vi "ADIS16448 Loop Inc Acquire Count.vi"(8 "error in (no error)":errorcluster) -> (0 "error out":errorcluster)   [LabVIEW 2019]
uses:
  ADIS16448 Globals.vi
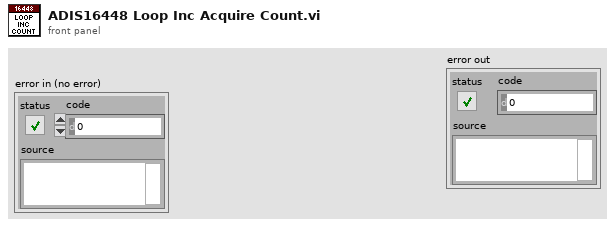
[diagram p1: front panel]
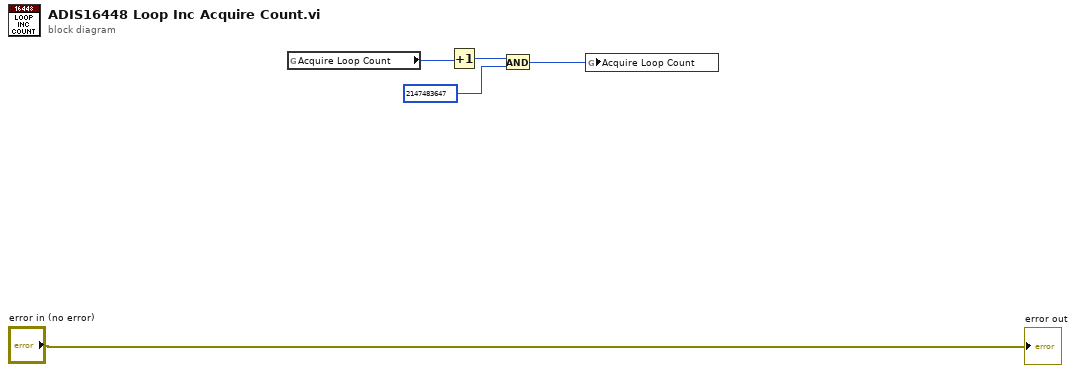
[diagram p0: block diagram]
diagram:
  n1 = global read "ADIS16448 Globals.vi" "Acquire Loop Count"() -> (w4:i32)
  n2 = Increment(x=w4) -> (x+1=w3:i32)
  n3 = And(x=w3, y=2147483647) -> (x .and. y?=w2:i32)
  n4 = global write "ADIS16448 Globals.vi" "Acquire Loop Count"(w2) -> ()
  "error out" <- "error in (no error)"
